vi "FromRepo.vi"(8 "error in":errorcluster, 9 "from repo cluster":T2, 10 "repository in":refnum<class "NISE_CEF_Repository.lvclass">, 11 "StepNode in":refnum<class "StepNode.lvclass">) -> (0 "error out":errorcluster, 2 "repository out":refnum<class "NISE_CEF_Repository.lvclass">, 3 "node":T1)   [LabVIEW 2015, in "StepNode.lvclass"]
doc: "Copyright 2017 National Instruments Corporation\n\nLicensed under the Apache License, Version 2.0 (the \"License\"); you may not use this file except in compliance with the License. You may obtain a copy of the License at http://www.apache.org/licenses/LICENSE-2.0\nUnless required by applicable law or agreed to in writing, software distributed under the License is distributed on an \"AS IS\" BASIS, WITHOUT WARRANTIES OR CONDITIONS OF ANY KIND, either express or implied. See the License for the specific language governing permissions and limitations under the License."
uses:
  StepNode.lvclass
  <vilib>/NI/Configuration Framework/Repository/NISE_CEF_Repository.lvclass
  <vilib>/NI/Configuration Framework/Node/FromRepoCluster.ctl
  <vilib>/NI/Configuration Framework/Node/NodeRef.ctl
  <vilib>/NI/Configuration Framework/Node/NISE_CEF_Node.lvclass
  SequenceRepo/SequenceRepo.lvclass
  StepNode.lvclass/StepNode.ctl
  Prototype/classes/Sequence/Config/Sequence Config.lvclass
  Prototype/classes/Step/Config/Step Config.lvclass
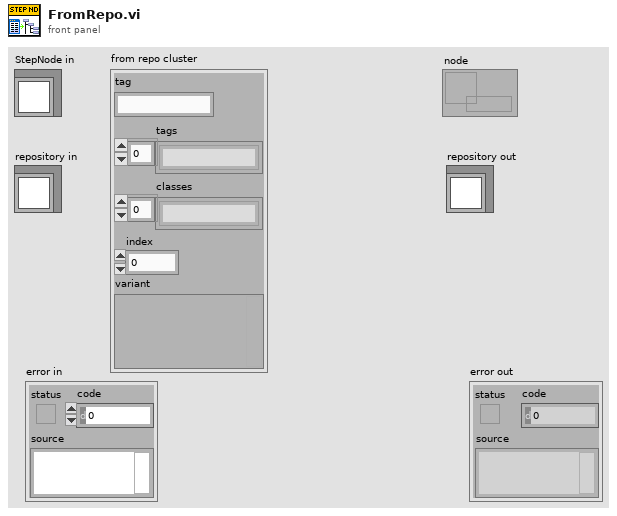
[diagram p1: front panel]
types:
  T1 = typedef "NISE_CEF_Node.lvclass/NodeRef.ctl" = refnum<data-value>
  T2 = typedef "NISE_CEF_Node.lvclass/FromRepoCluster.ctl" = cluster{"tag":string, "tags":string[], "classes":string[], "index":i32, "variant":variant}
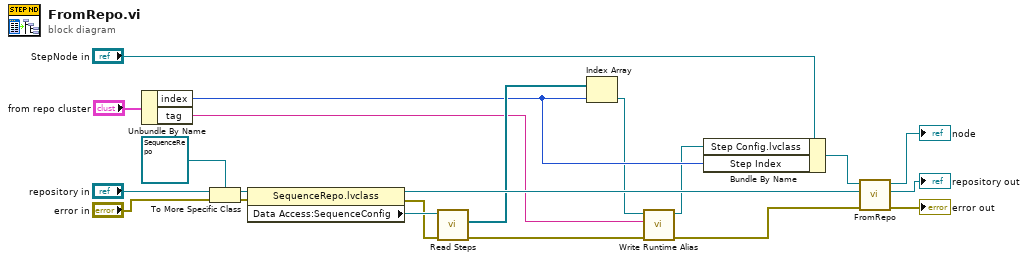
[diagram p0: block diagram]
diagram:
  n1 = Unbundle By Name("from repo cluster") -> ("index"=w5:i32, "tag"=w1:string)
  n2 = To More Specific Class(target class=refnum<class "SequenceRepo.lvclass"> refnum ("cRIO repo.lvclass"), reference="repository in", error in="error in") -> (specific class reference=w13:refnum<class "SequenceRepo.lvclass">, error out=w9:errorcluster)
  n3 = property class="SequenceRepo.lvclass"(reference=w13, error in=w9) -> (reference out=w12:refnum<class "SequenceRepo.lvclass">, error out=w7:errorcluster, "Data Access:SequenceConfig"=w11:refnum<class "Sequence Config.lvclass">)
  n4 = call-dynamic "Read Steps.vi"("error in (no error)"=w7, "Sequence in"=w11) -> ("error out"=w6:errorcluster, "Steps"=w8:refnum<class "Step Config.lvclass">[])  [unwired: 7 in, 1 out]
  n5 = Index Array(array=w8, index=w5) -> (element=w3:refnum<class "Step Config.lvclass">)
  n6 = call-dynamic "Write Runtime Alias.vi"("error in (no error)"=w6, "Runtime Alias"=w1, "Step Config in"=w3) -> ("error out"=w4:errorcluster, "Step Config out"=w2:refnum<class "Step Config.lvclass">)  [unwired: 7 in]
  n7 = Bundle By Name(cluster="StepNode in", "Step Config.lvclass"=w2, "Step Index"=w5) -> (w17:refnum<class "StepNode.lvclass">)
  n8 = call-parent "FromRepo.vi"("error in"=w4, "repository in"=w12, "node in"=w17) -> ("error out"=→"error out":errorcluster, "repository out"=→"repository out":refnum<class "NISE_CEF_Repository.lvclass">, "node"=→"node":T1)  [unwired: 6 in]
